vi "Configure Measurement Filter.vi"(6 "Filter Count (1)":i32=1, 7 "Filter Type (0: Moving Average Filter)":i32(ring) items=["Moving Average Filter ", "Repeat Filter", "Median Filter"], 8 "error in (no error)":errorcluster, 9 "Enable Filter (F: Disable)":bool, 10 "Source Measure Unit Channel (0: Channel A)":i32(ring) items=["Channel A", "Channel B"], 11 "VISA resource name":refnum<visa-resource-name>) -> (0 "error out":errorcluster, 3 "VISA resource name out":refnum<visa-resource-name>)   [LabVIEW 2020, in "Keithley 2600 Series.lvlib"]
doc: "Configures the measurement filter."
uses:
  <instrlib>/Keithley 2600 Series/Keithley 2600 Series.lvlib
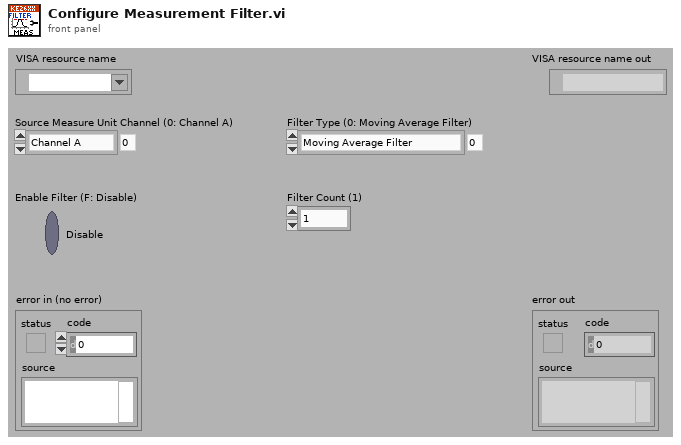
[diagram p1: front panel]
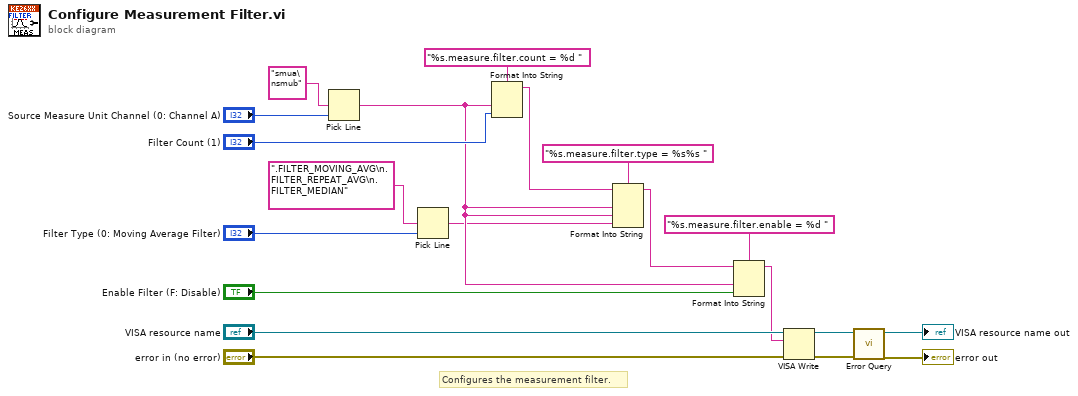
[diagram p0: block diagram]
diagram:
  # "Configures the measurement filter."
  n1 = Pick Line(multi-line string="smua\nsmub", line index="Source Measure Unit Channel (0: Channel A)") -> (output string=w6:string)  [unwired: 1 in]
  n2 = Pick Line(multi-line string=".FILTER_MOVING_AVG\n.FILTER_REPEAT_AVG\n.FILTER_MEDIAN", line index="Filter Type (0: Moving Average Filter)") -> (output string=w5:string)  [unwired: 1 in]
  n3 = Format Into String(format string="%s.measure.filter.count = %d ", w6, "Filter Count (1)") -> (resulting string=w4:string)  [unwired: 2 in, 1 out]
  n4 = Format Into String(format string="%s.measure.filter.type = %s%s ", initial string=w4, w6, w6, w5) -> (resulting string=w2:string)  [unwired: 1 in, 1 out]
  n5 = Format Into String(format string="%s.measure.filter.enable = %d ", initial string=w2, w6, "Enable Filter (F: Disable)") -> (resulting string=w3:string)  [unwired: 1 in, 1 out]
  n6 = VISA Write(VISA resource name="VISA resource name", write buffer=w3, error in (no error)="error in (no error)") -> (VISA resource name out=w14:refnum<visa-resource-name>, error out=w13:errorcluster)  [unwired: 1 out]
  n7 = call <instrlib>:"Error Query.vi"("error in (no error)"=w13, "VISA resource name"=w14) -> ("error out"=→"error out":errorcluster, "VISA resource name out"=→"VISA resource name out":refnum<visa-resource-name>)  [unwired: 6 in, 2 out]
